vi "FPGA Read Array - U32.vi"(8 "error in (no error)":errorcluster, 10 "Indicator":T1, 11 "FPGA Session In":refnum<class "Firmware Independent PID Interface.lvclass">) -> (0 "error out":errorcluster, 2 "Array":u32[](array[numeric]), 3 "FPGA Session Out":refnum<class "Firmware Independent PID Interface.lvclass">)   [LabVIEW 2010, in "Firmware Independent PID Interface.lvclass"]
doc: "Reads an entire array of unsigned 32-bit integer values from a given array indicator or control."
uses:
  Firmware Independent PID Interface.lvclass
  TypeDefs/IndicatorArrayU32.ctl
  <vilib>/rvi/DataTransferAndStorage/Container/Common/niFpgaDataTypeControl.ctl
  <userlib>/_FPGA Interface Advanced Tools/FPGA Interface Base/FPGA Interface Base.lvclass/FPGA Interface Base.ctl
  <vilib>/Utility/error.llb/Error Cluster From Error Code.vi
  <userlib>/_FPGA Interface Advanced Tools/FPGA Interface Base/Accessors/FPGA Read Session.vi
  <userlib>/_FPGA Interface Advanced Tools/FPGA Interface Wrapper/FPGA Interface Wrapper.lvlib
  <userlib>/_FPGA Interface Advanced Tools/FPGA Interface Base/FPGA Interface Base.lvclass
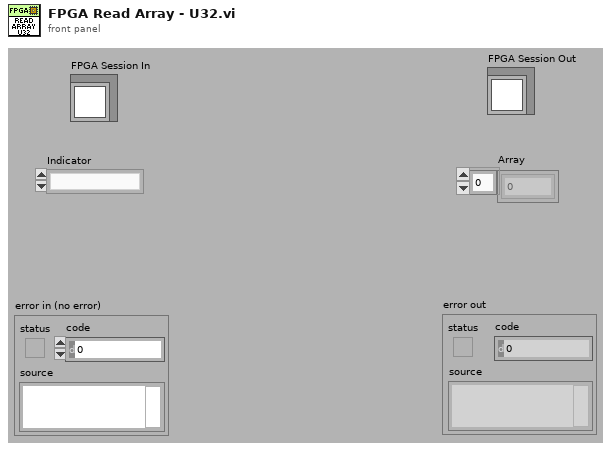
[diagram p1: front panel]
types:
  T1 = typedef "Firmware Independent PID Interface.lvclass/IndicatorArrayU32.ctl" = enum16{""}
  T2 = typedef "niFpgaDataTypeControl.ctl" = enum32{"Boolean", "I8", "I16", "I32", "I64", "U8", "U16", "U32", "U64", "FXP", "CustomControl"}
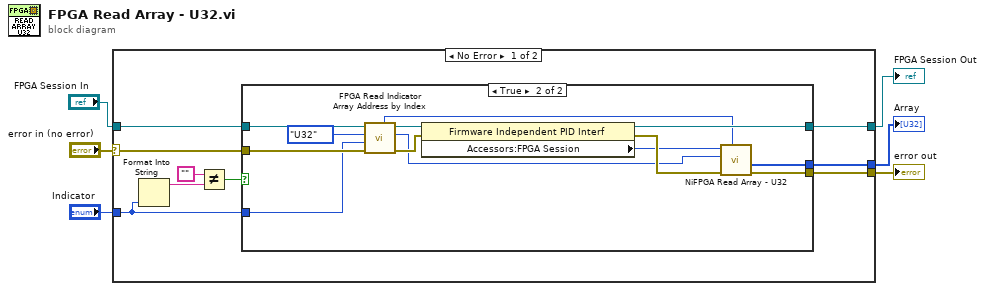
[diagram p0: block diagram]
diagram:
  n1 = case shown="No Error" "error in (no error)" {
    selector: "error in (no error)" -> [w7 w32]
    tunnel: [w10 w32] -> w1
    tunnel: [w8 w31] -> w3
    tunnel: [w9 _] -> w2
    tunnel: "FPGA Session In" -> [w13 w31]
    tunnel: "Indicator" -> [w11 _]
    frame No Error {
      n2 = Format Into String(w11) -> (resulting string=w15:string)  [unwired: 3 in, 1 out]
      n3 = Not Equal?(x="", y=w15) -> (x != y?=w12:bool)
      n4 = case shown="True" w12 {
        tunnel: [w16 w22] -> w10
        tunnel: [w17 w26] -> w8
        tunnel: [_ w21] -> w9
        tunnel: w13 -> [w17 w27]
        tunnel: w11 -> [_ w24]
        tunnel: w7 -> [w16 w25]
        frame False {
        }
        frame True {
          n5 = call <userlib>:"FPGA Read Indicator Array Address by Index.vi"("error in (no error)"=w25, "index"=w24, "Data Type"=niFpgaDataTypeControl."U32", "FPGA Interface Base in"=w27) -> ("error out"=w29:errorcluster, "Address"=w20:u32, "FPGA Interface Base out"=w28:refnum<class "Firmware Independent PID Interface.lvclass">, "Num Elements"=w18:u32)  [unwired: 3 in, 1 out]
          n6 = property class="Firmware Independent PID Interf"(reference=w28, error in=w29) -> (reference out=w26:refnum<class "Firmware Independent PID Interface.lvclass">, error out=w23:errorcluster, "Accessors:FPGA Session"=w19:u32)
          n7 = call <userlib>:"NiFPGA Read Array - U32.vi"("Size"=w18, "error in (no error)"=w23, "Indicator"=w20, "Session"=w19) -> ("error out"=w22:errorcluster, "Array"=w21:u32[])  [unwired: 5 in, 1 out]
        }
      }
    }
    frame Error {
    }
  }
  "error out" <- w1
  "FPGA Session Out" <- w3
  "Array" <- w2
